vi "Data_CalReadCount.vi"(9 "显示长度":i32, 10 "采样长度":i32) -> (1 "显示段数":i32[](array[numeric]))   [LabVIEW 2013]
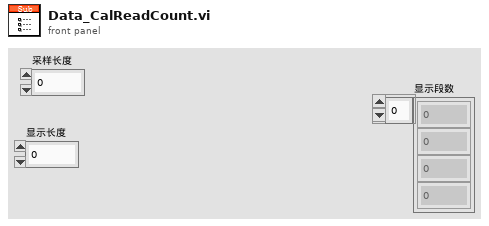
[diagram p1: front panel]
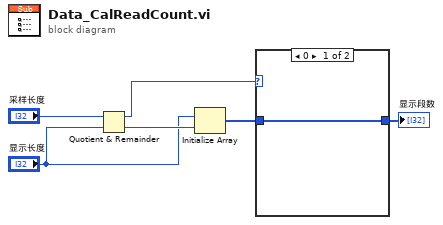
[diagram p0: block diagram]
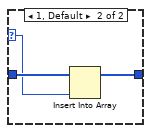
[diagram p2: hidden frame]
diagram:
  n1 = Quotient & Remainder(x="采样长度", y="显示长度") -> (x-y*floor(x/y)=w3:i32, floor(x/y)=w5:i32)
  n2 = Initialize Array("显示长度", w5) -> (w2:i32[])
  n3 = case shown="0" w3 {
    selector: w3 -> [_ w9]
    tunnel: w2 -> [w7 w10]
    tunnel: [w7 w8] -> w1
    frame 0 {
    }
    frame 1, Default {
      n4 = Insert Into Array(array=w10, new element=w9) -> (w8:i32[])  [unwired: 1 in]
    }
  }
  "显示段数" <- w1
